vi "Main-Basic.vi"() -> ()   [LabVIEW 2019]
uses:
  Device.Simulation/Device.Simulation/Device.Simulation.lvclass
  C:/Repos/KLA-Demo/Source/Subsystems/BASE/BASE/BASE.lvclass
  D:/Program Files (x86)/National Instruments/LabVIEW 2019/vi.lib/ActorFramework/Actor/Actor.lvclass
  Subsystems/BASE.Device/BASE.Device/BASE.Device.lvclass
  <vilib>/ActorFramework/Message Enqueuer/Message Enqueuer.lvclass/Message Enqueuer.ctl
  <vilib>/ActorFramework/Message Enqueuer/Enqueue.vi
  <vilib>/ActorFramework/Stop Msg/Stop Msg.lvclass
  D:/Program Files (x86)/National Instruments/LabVIEW 2019/vi.lib/ActorFramework/Message/Message.lvclass
  <vilib>/ActorFramework/Message Priority Queue/Priority Enqueue.vi
  <vilib>/ActorFramework/Actor/Actor.lvclass
  Subsystems/BASE/BASE/BASE.lvclass
panel:
  in  "Stop":bool
  in  "config file path (Empty: use configured)":path
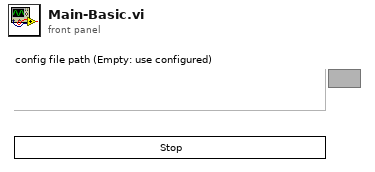
[diagram p1: front panel]
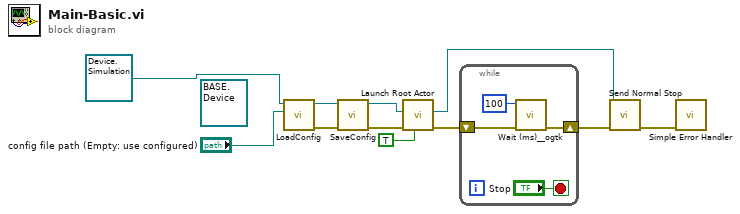
[diagram p0: block diagram]
diagram:
  (unwired) refnum<class "BASE.Device.lvclass"> refnum ("BASE.Device.lvlib:BASE.Device.lvclass")
  n1 = call "LoadConfig.vi"("config file path (Empty: use configured)"="config file path (Empty: use configured)", "BASE in"=refnum<class "Device.Simulation.lvclass"> refnum ("Device.Simulation.lvlib:Device.Simulation.lvclass")) -> ("error out"=w7:errorcluster, "BASE out"=w10:refnum<class "Device.Simulation.lvclass">)  [unwired: 8 in]
  n2 = call "SaveConfig.vi"("error in (no error)"=w7, "BASE in"=w10) -> ("error out"=w6:errorcluster, "BASE out"=w5:refnum<class "Device.Simulation.lvclass">)  [unwired: 8 in]
  n3 = call <vilib>:"Launch Root Actor.vi"("Open Actor Core front panel? (F)"=TRUE, "error in (no error)"=w6, "Actor"=w5) -> ("error out"=w4:errorcluster, "Actor's Enqueuer"=w9:refnum<class "Message Enqueuer.lvclass">)  [unwired: 7 in]
  n4 = while {
    shift-right: [w14] -> w2
    shift-left: w4 -> [w15]
    stop <- "Stop" stop-if-true
    n5 = call <userlib>:"Wait (ms)__ogtk.vi"("error in (no error)"=w15, "milliseconds to wait"=u32 100) -> ("error out"=w14:errorcluster)  [unwired: 8 in, 1 out]
  }
  n6 = call <vilib>:"Send Normal Stop.vi"("error in (no error)"=w2, "Message Enqueuer"=w9) -> ("error out"=w3:errorcluster)  [unwired: 9 in]
  n7 = call <vilib>:"Simple Error Handler.vi"("error in (no error)"=w3) -> ()  [unwired: 4 in, 5 out]
